vi "classifier.vi"(5 "existingTarget":bool, 6 "ImageSize":cluster{"Width":u32, "Height":u32}, 7 "targetCount":i32, 8 "input array":T2(array[cluster]), 9 "data":string, 10 "InitialValues":i32[](array[numeric]), 11 "Image In":T1(plugin-control)) -> (0 "output array":T2(array[cluster]))   [LabVIEW 2014]
uses:
  <vilib>/vision/Image Controls.llb/IMAQ Image.ctl
  <vilib>/vision/NI_Vision_Development_Module.lvlib
panel:
  out "cancelled?":bool=TRUE
  out "index":u32
  in  "numLocations":i32
  out "pitch":dbl
  out "roll":dbl
  out "yaw":dbl
  out "aircraftAltitude":dbl
  out "aircraftLongitude":dbl format="%#_10g"
  out "aircrftLatitude":dbl format="%#_10g"
  out "dragStart":cluster{"X":i32, "Y":i32}
  out "state":i32
  in  "Longitude":dbl format="%#_10g"
  in  "Latitude":dbl format="%#_10g"
  in  "changeOrientation":bool
  in  "Orientation":u16(ring) items=["North", "North-East", "East", "South-East", "South", "South-West", "West", "North-West"]
  in  "done":bool
  in  "Alphanumeric Color":string
  in  "Alphanumeric":string
  in  "Background Color":string
  in  "Shape":string
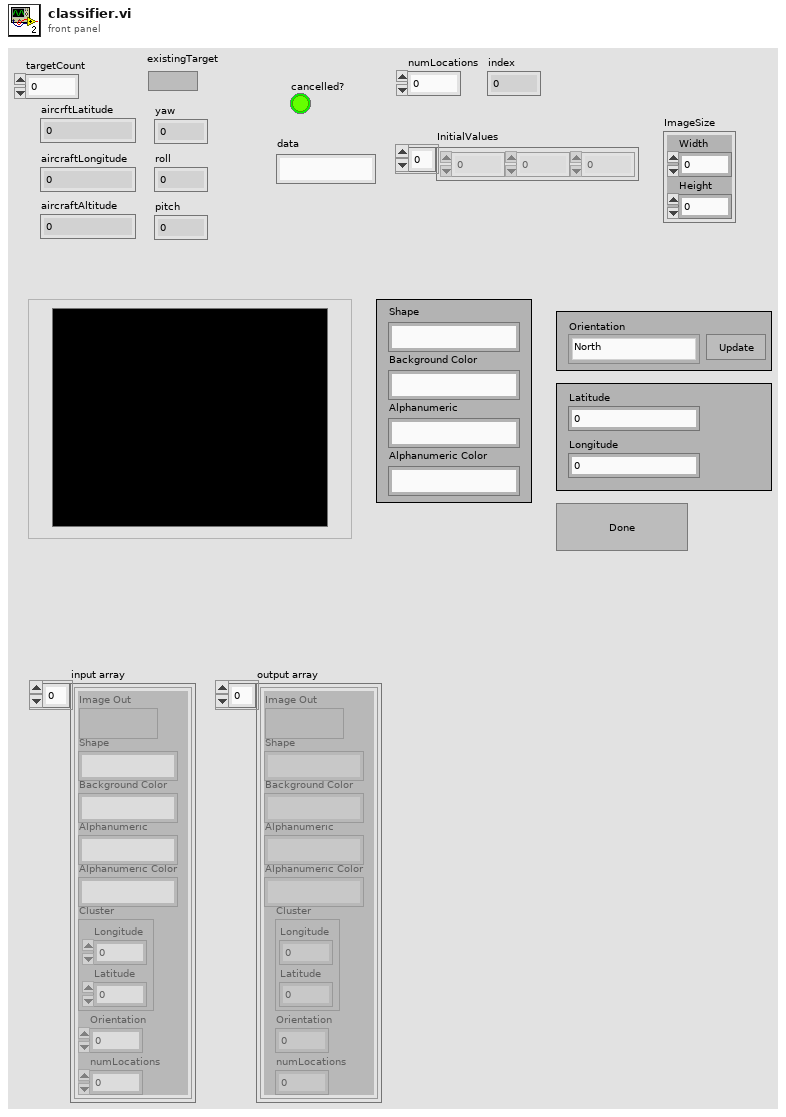
[diagram p1: front panel]
types:
  T1 = typedef "IMAQ Image.ctl" = refnum<image>
  T2 = cluster{"Image Out":T1, "Shape":string, "Background Color":string, "Alphanumeric":string, "Alphanumeric Color":string, "Cluster":cluster{"Longitude":dbl, "Latitude":dbl}, "Orientation":u16, "numLocations":i32}[]
  T3 = cluster{"Global Rectangle":i32[], "Contours":cluster{"Contour Type":u32, "ROI Type":u32, "Points":i32[]}[]}
  T4 = cluster{"Image Out":T1, "Shape":string, "Background Color":string, "Alphanumeric":string, "Alphanumeric Color":string, "Cluster":cluster{"Longitude":dbl, "Latitude":dbl}, "Orientation":u16, "numLocations":i32}
  T5 = typedef "Image Type" = u32
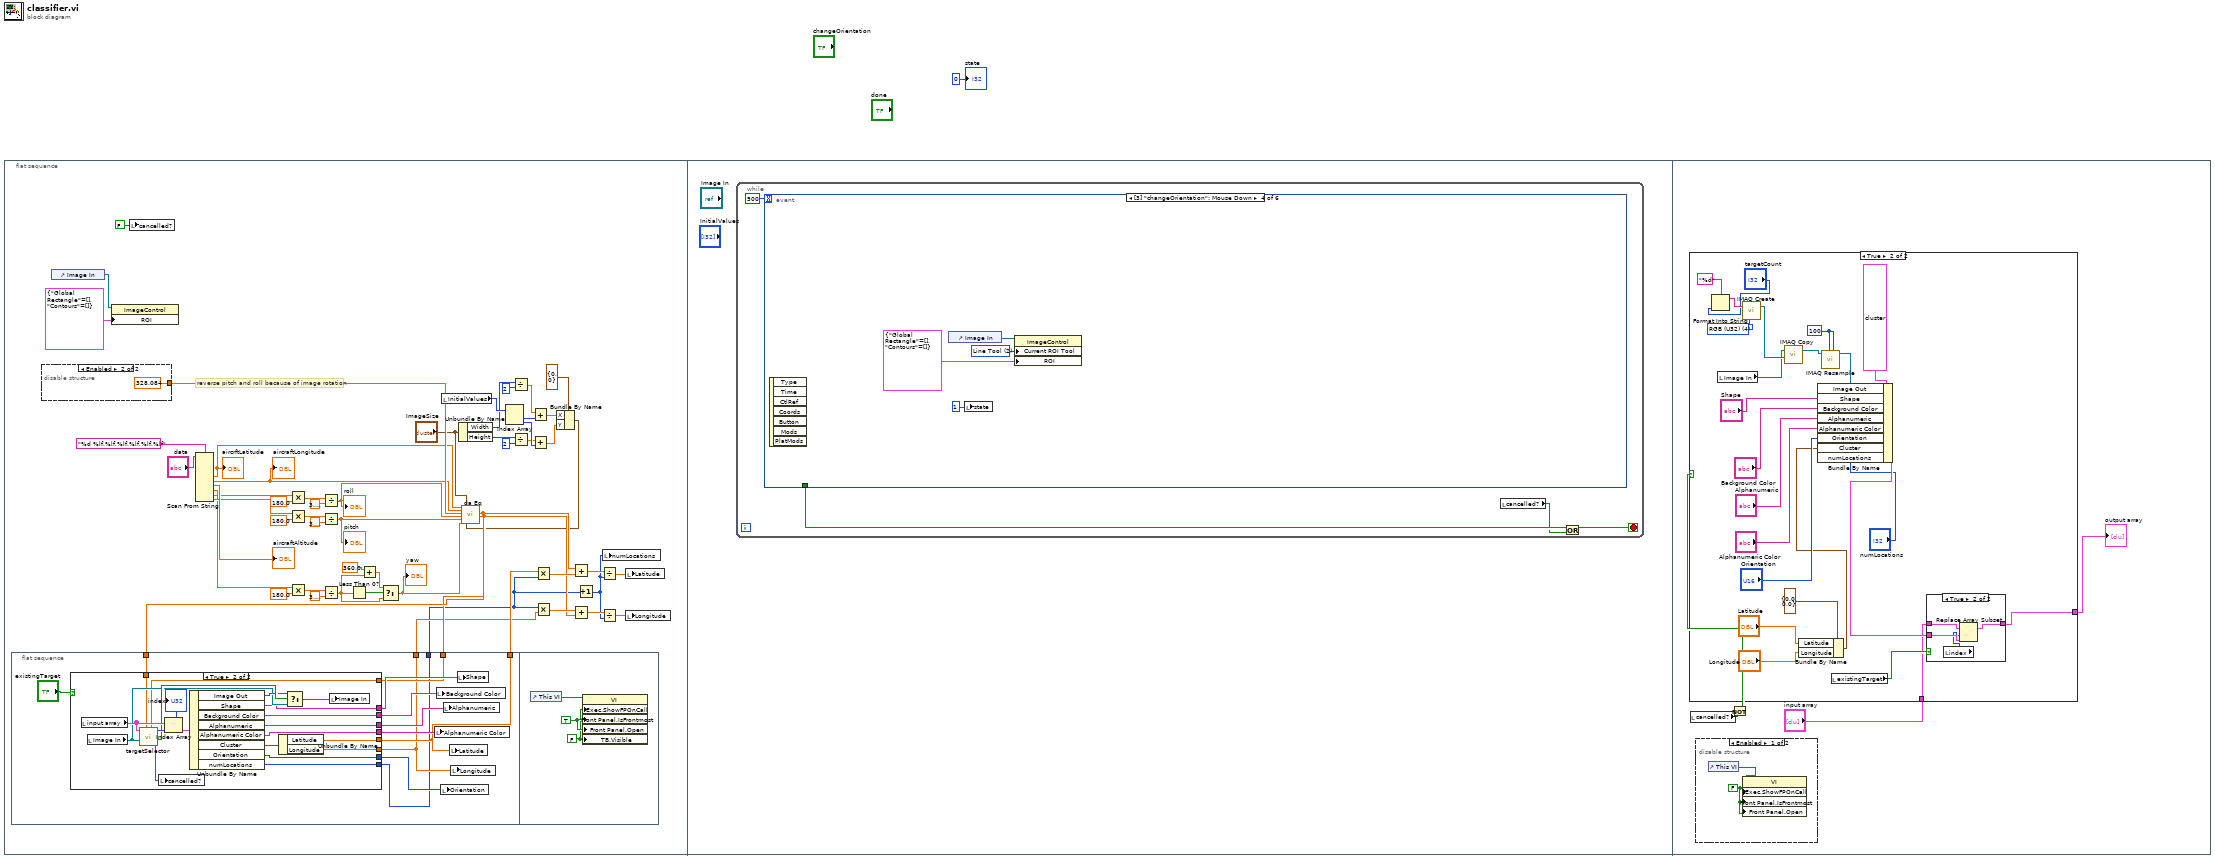
[diagram p0: block diagram]
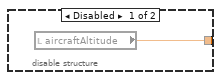
[diagram p2: hidden frame]
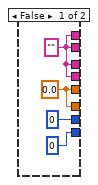
[diagram p3: hidden frame]
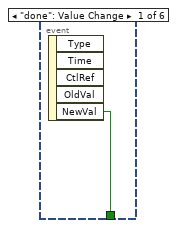
[diagram p4: hidden frame]
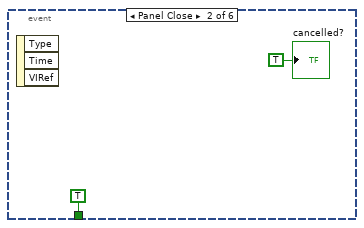
[diagram p5: hidden frame]
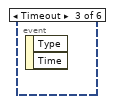
[diagram p6: hidden frame]
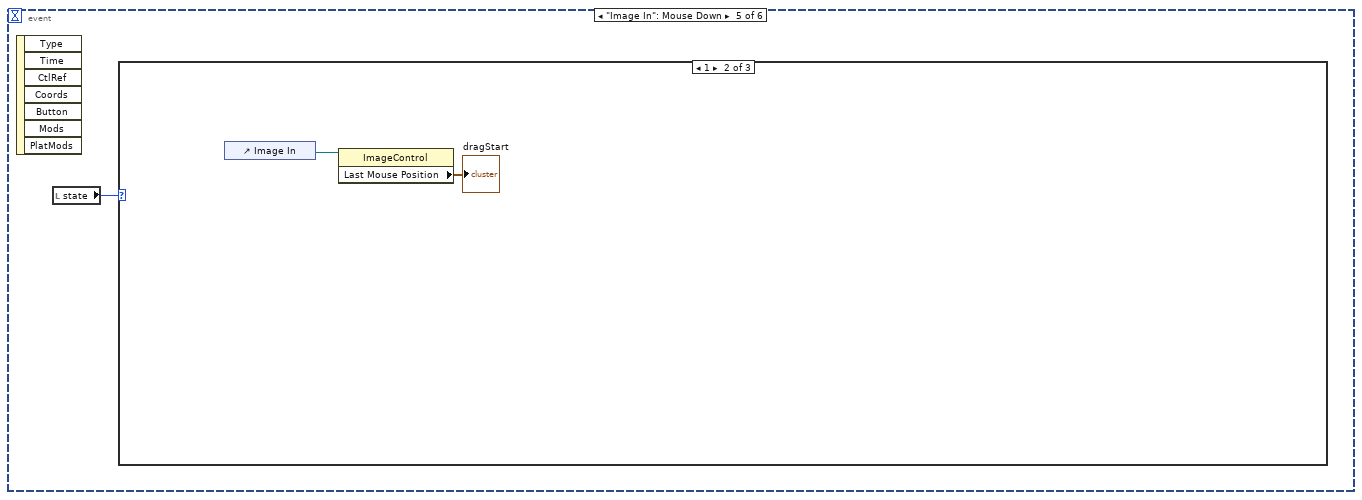
[diagram p7: hidden frame]
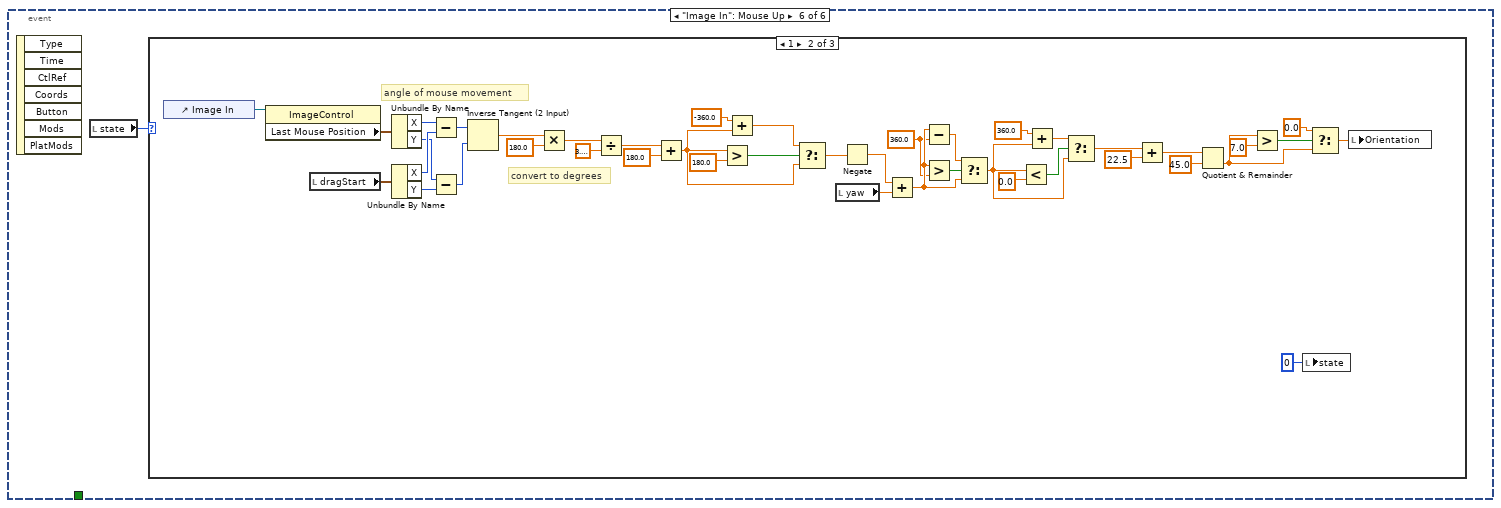
[diagram p10: hidden frame]
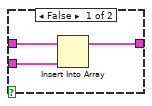
[diagram p14: hidden frame]
diagram:
  n1 = flat-sequence {
    frame #0 {
      # "reverse pitch and roll because of image rotation"
      n2 = flat-sequence {
        tunnel: w8 -> [w62]
        tunnel: w7 -> [w61]
        tunnel: [w60] -> w4
        tunnel: [w59] -> w3
        tunnel: [w58] -> w2
        frame #0 {
          n3 = case shown="True" "existingTarget" {
            tunnel: [w72 w84] -> w67
            tunnel: [w72 w83] -> w66
            tunnel: [w72 w82] -> w65
            tunnel: [w72 w81] -> w64
            tunnel: [w71 w79] -> w60
            tunnel: [w71 w78] -> w59
            tunnel: [u16 0 ("Orientation") w77] -> w63
            tunnel: [0 ("numLocations") w76] -> w58
            tunnel: w62 -> [_ w75]
            tunnel: w61 -> [_ w74]
            frame False {
              w71 = 0.0 ("Latitude")
              w72 = "" ("Shape")
            }
            frame True {
              n4 = local read "input array"() -> (w91:T2)
              n5 = local read "Image In"() -> (w86:T1)
              n6 = call "targetSelector.vi"("Longitude"=w74, "Latitude"=w75, "New Target"=w86, "Existing Targets"=w91) -> ("cancelled"=w73:bool, "imageSelect 2"=w88:bool, "index"=w90:u32)  [unwired: 5 in]
              "index" <- w90
              n7 = local write "cancelled?"(w73) -> ()
              n8 = Index Array(array=w91, index=w90) -> (element=w89:T4)
              n9 = Unbundle By Name(w89) -> ("Image Out"=w87:T1, "Shape"=w84:string, "Background Color"=w83:string, "Alphanumeric"=w82:string, "Alphanumeric Color"=w81:string, "Cluster"=w80:cluster{"Longitude":dbl, "Latitude":dbl}, "Orientation"=w77:u16, "numLocations"=w76:i32)
              n10 = Unbundle By Name(w80) -> ("Latitude"=w79:dbl, "Longitude"=w78:dbl)
              n11 = Select(t=w87, s=w88, f=w86) -> (s? t:f=w85:T1)
              n12 = local write "Image In"(w85) -> ()
            }
          }
          n13 = local write "Alphanumeric Color"(w64) -> ()
          n14 = local write "Background Color"(w66) -> ()
          n15 = local write "Orientation"(w63) -> ()
          n16 = local write "Alphanumeric"(w65) -> ()
          n17 = local write "Latitude"(w60) -> ()
          n18 = local write "Longitude"(w59) -> ()
          n19 = local write "Shape"(w67) -> ()
        }
        frame #1 {
          w92 = FALSE ("Tool Bar:Visible")
          w94 = TRUE ("Execution:Show Front Panel On Call")
          n20 = control-ref of="This VI"() -> (w93:refnum<vi>)
          n21 = property class="VI"(reference=w93, "Exec.ShowFPOnCall"=w92, "Front Panel.IsFrontmost"=w94, "Front Panel.Open"=w94, "TB.Visible"=w92) -> ()  [unwired: 1 in, 2 out]
        }
      }
      n22 = disable-structure shown="Enabled" {
        disable-tunnel: [w56 328.084 ("Plane Height (ft)")] -> w33
        frame Disabled {
          n23 = local read "aircraftAltitude"() -> (w56:dbl)
        }
        frame Enabled {
        }
      }
      n24 = control-ref of="Image In"() -> (w36:refnum<vi>)
      n25 = property class="ImageControl"(reference=w36, "ROI"=T3 {"Global Rectangle"=[], "Contours"=[]}) -> ()  [unwired: 1 in, 2 out]
      n26 = local write "cancelled?"(FALSE ("cancelled?")) -> ()
      n27 = Scan From String(format string="%d %lf,%lf,%lf,%lf,%lf,%lf", input string="data") -> (output 2=w17:dbl, output 3=w16:dbl, output 4=→"aircraftAltitude":dbl, output 5=w45:dbl, output 6=w41:dbl, output 7=w49:dbl)  [unwired: 10 in, 3 out]
      "aircrftLatitude" <- w17
      "aircraftLongitude" <- w16
      n28 = Multiply(x=w41, y=180.0) -> (x*y=w43:dbl)
      n29 = Multiply(x=w49, y=180.0) -> (x*y=w51:dbl)
      n30 = Multiply(x=w45, y=180.0) -> (x*y=w47:dbl)
      n31 = Divide(x=w43, y=3.141592653589793) -> (x/y=w20:dbl)
      "roll" <- w20
      n32 = Divide(x=w51, y=3.141592653589793) -> (x/y=w19:dbl)
      "pitch" <- w19
      n33 = Divide(x=w47, y=3.141592653589793) -> (x/y=w39:dbl)
      n34 = Less Than 0?(x=w39) -> (x < 0?=w40:bool)
      n35 = Add(x=360.0, y=w39) -> (x+y=w37:dbl)
      n36 = Select(t=w37, s=w40, f=w39) -> (s? t:f=w18:dbl)
      "yaw" <- w18
      n37 = local read "InitialValues"() -> (w30:i32[])
      n38 = Unbundle By Name("ImageSize") -> ("Width"=w14:u32, "Height"=w13:u32)
      n39 = Index Array(array=w30) -> (element #1=w29:i32, element #2=w28:i32)  [unwired: 2 in]
      n40 = Divide(x=w14, y=u32 2) -> (x/y=w10:dbl)
      n41 = Divide(x=w13, y=u32 2) -> (x/y=w9:dbl)
      n42 = Add(x=w10, y=w29) -> (x+y=w32:dbl)
      n43 = Add(x=w9, y=w28) -> (x+y=w31:dbl)
      n44 = Multiply(x=w4, y=w2) -> (x*y=w27:dbl)
      n45 = Multiply(x=w2, y=w3) -> (x*y=w26:dbl)
      n46 = Bundle By Name(cluster=cluster{"X":i32, "Y":i32} {"X"=0, "Y"=0} ("Last Mouse Position:All Elements"), "X"=w32, "Y"=w31) -> (w5:cluster{"X":i32, "Y":i32})
      n47 = call "da Eq.vi"("Plane Lat"=w17, "Plane Lon"=w16, "Plane Height (ft)"=w33, "Plane Roll"=w20, "Plane Pitch"=w19, "Plane Heading"=w18, "Displayed Image:Size:All Elements"="ImageSize", "Last Mouse Position:All Elements"=w5) -> ("Latitude"=w8:dbl, "Longitude"=w7:dbl)  [unwired: 10 in]
      n48 = Add(x=w8, y=w27) -> (x+y=w24:dbl)
      n49 = Add(x=w26, y=w7) -> (x+y=w25:dbl)
      n50 = Increment(x=w2) -> (x+1=w23:i32)
      n51 = Divide(x=w24, y=w23) -> (x/y=w22:dbl)
      n52 = Divide(x=w25, y=w23) -> (x/y=w21:dbl)
      n53 = local write "numLocations"(w23) -> ()
      n54 = local write "Latitude"(w22) -> ()
      n55 = local write "Longitude"(w21) -> ()
    }
    frame #1 {
      n56 = while {
        stop <- w96 stop-if-true
        n57 = event shown="[3] \"changeOrientation\": Mouse Down" {
          selector: _ -> [_ _ _ _ _ _]
          dyn-events: _ -> [_ _ _ _ _ _]
          timeout: 500 -> [_ _ _ _ _ _]
          tunnel: [w99 TRUE ("NewVal") _ _ _ _] -> w98
          event "done": Value Change {
            n58 = event-data() -> ("NewVal"=w99:bool)  [unwired: 1 in, 4 out]
          }
          event Panel Close {
            n59 = event-data() -> ()  [unwired: 1 in, 3 out]
            "cancelled?" <- TRUE
          }
          event Timeout {
            n60 = event-data() -> ()  [unwired: 1 in, 2 out]
          }
          event "changeOrientation": Mouse Down {
            w104 = u32 2 items=["Zoom Tool"=8, "Selection Tool"=0, "Pan Tool"=9, "Point Tool"=1, "Line Tool"=2, "Rectangle Tool"=3, "Rotated Rectangle Tool"=12, "Polyline Tool"=10, "Polygon Tool"=5, "Freehand Tool"=11, "Closed Freehand Tool"=6, "Ellipse Tool"=4, "Annulus Tool"=7] ("Current ROI Tool")
            n61 = event-data() -> ()  [unwired: 1 in, 7 out]
            n62 = control-ref of="Image In"() -> (w105:refnum<vi>)
            n63 = local write "state"(1 ("state")) -> ()
            n64 = property class="ImageControl"(reference=w105, "Current ROI Tool"=w104, "ROI"=T3 {"Global Rectangle"=[], "Contours"=[]}) -> ()  [unwired: 1 in, 2 out]
          }
          event "Image In": Mouse Down {
            n65 = event-data() -> ()  [unwired: 1 in, 7 out]
            n66 = local read "state"() -> (w106:i32)
            n67 = case shown="1" w106 {
              frame 0, Default {
              }
              frame 1 {
                n68 = control-ref of="Image In"() -> (w108:refnum<vi>)
                n69 = property class="ImageControl"(reference=w108) -> ("Last Mouse Position"=→"dragStart":cluster{"X":i32, "Y":i32})  [unwired: 1 in, 2 out]
              }
              frame 2 {
              }
            }
          }
          event "Image In": Mouse Up {
            n70 = event-data() -> ()  [unwired: 1 in, 7 out]
            n71 = local read "state"() -> (w109:i32)
            n72 = case shown="1" w109 {
              frame 0, Default {
              }
              frame 1 {
                w127 = 360.0 ("y")
                # "convert to degrees"
                # "angle of mouse movement"
                n73 = control-ref of="Image In"() -> (w145:refnum<vi>)
                n74 = property class="ImageControl"(reference=w145) -> ("Last Mouse Position"=w144:cluster{"X":i32, "Y":i32})  [unwired: 1 in, 2 out]
                n75 = local read "dragStart"() -> (w143:cluster{"X":i32, "Y":i32})
                n76 = Unbundle By Name(w144) -> ("X"=w142:i32, "Y"=w139:i32)
                n77 = Unbundle By Name(w143) -> ("X"=w141:i32, "Y"=w140:i32)
                n78 = Subtract(x=w142, y=w141) -> (x-y=w151:i32)
                n79 = Subtract(x=w139, y=w140) -> (x-y=w150:i32)
                n80 = Inverse Tangent (2 Input)(1:w150, 2:w151) -> (0:w149:dbl)
                n81 = Multiply(x=w149, y=180.0) -> (x*y=w147:dbl)
                n82 = Divide(x=w147, y=3.141592653589793) -> (x/y=w138:dbl)
                n83 = Add(x=w138, y=180.0) -> (x+y=w134:dbl)
                n84 = Greater?(x=w134, y=180.0) -> (0:w135:bool)
                n85 = Add(x=-360.0, y=w134) -> (x+y=w132:dbl)
                n86 = Select(t=w132, s=w135, f=w134) -> (s? t:f=w131:dbl)
                n87 = local read "yaw"() -> (w130:dbl)
                n88 = Negate(x=w131) -> (-x=w125:dbl)
                n89 = Add(x=w125, y=w130) -> (x+y=w128:dbl)
                n90 = Subtract(x=w128, y=w127) -> (x-y=w126:dbl)
                n91 = Greater?(x=w128, y=w127) -> (0:w129:bool)
                n92 = Select(t=w126, s=w129, f=w128) -> (s? t:f=w122:dbl)
                n93 = Less?(x=w122, y=0.0) -> (x < y?=w123:bool)
                n94 = Add(x=360.0, y=w122) -> (x+y=w120:dbl)
                n95 = Select(t=w120, s=w123, f=w122) -> (s? t:f=w119:dbl)
                n96 = Add(x=w119, y=22.5) -> (x+y=w117:dbl)
                n97 = Quotient & Remainder(x=w117, y=45.0) -> (floor(x/y)=w113:dbl)  [unwired: 1 out]
                n98 = Greater?(x=w113, y=7.0) -> (0:w114:bool)
                n99 = local write "state"(0 ("state")) -> ()
                n100 = Select(t=0.0, s=w114, f=w113) -> (s? t:f=w111:dbl)
                n101 = local write "Orientation"(w111) -> ()
              }
              frame 2 {
              }
            }
          }
        }
        n102 = local read "cancelled?"() -> (w95:bool)
        n103 = Or(x=w98, y=w95) -> (x .or. y?=w96:bool)
      }
    }
    frame #2 {
      n104 = local read "cancelled?"() -> (w155:bool)
      n105 = disable-structure shown="Enabled" {
        frame Enabled {
          w189 = FALSE ("Execution:Show Front Panel On Call")
          n106 = control-ref of="This VI"() -> (w188:refnum<vi>)
          n107 = property class="VI"(reference=w188, "Exec.ShowFPOnCall"=w189, "Front Panel.IsFrontmost"=w189, "Front Panel.Open"=w189) -> ()  [unwired: 1 in, 2 out]
        }
        frame Disabled {
        }
      }
      n108 = Not(x=w155) -> (.not. x?=w154:bool)
      n109 = case shown="True" w154 {
        tunnel: [w156 w158] -> w153
        tunnel: "input array" -> [w156 w157]
        frame False {
        }
        frame True {
          w162 = 100
          w169 = T5 4 items=["Grayscale (U8)", "Grayscale (I16)", "Grayscale (SGL)", "Complex (CSG)", "RGB (U32)", "HSL (U32)", "RGB (U64)", "Grayscale (U16)"] ("Image Type")
          n110 = Format Into String(format string="%d", "targetCount") -> (resulting string=w166:string)  [unwired: 2 in, 1 out]
          n111 = local read "Image In"() -> (w167:T1)
          n112 = call "IMAQ Create"("Image Name"=w166, "Image Type"=w169) -> ("New Image"=w168:T1)  [unwired: 3 in, 1 out]
          n113 = call "IMAQ Copy"("Image Dst"=w168, "Image Src"=w167) -> ("Image Dst Out"=w163:T1)  [unwired: 4 in, 1 out]
          n114 = Bundle By Name(cluster=cluster{"Longitude":dbl, "Latitude":dbl} {"Longitude"=0.0, "Latitude"=0.0} ("Cluster"), "Latitude"="Latitude", "Longitude"="Longitude") -> (w172:cluster{"Longitude":dbl, "Latitude":dbl})
          n115 = call "IMAQ Resample"("X Resolution"=w162, "Y Resolution"=w162, "Image Src"=w163) -> ("Image Dst Out"=w161:T1)  [unwired: 7 in, 1 out]
          n116 = Bundle By Name(cluster=T4 {"Image Out"=refnum, "Shape"="", "Background Color"="", "Alphanumeric"="", "Alphanumeric Color"="", "Cluster"={"Longitude"=0.0, "Latitude"=0.0}, "Orientation"=0, "numLocations"=0} ("output cluster"), "Image Out"=w161, "Shape"="Shape", "Background Color"="Background Color", "Alphanumeric"="Alphanumeric", "Alphanumeric Color"="Alphanumeric Color", "Orientation"="Orientation", "Cluster"=w172, "numLocations"="numLocations") -> (w171:T4)
          n117 = local read "existingTarget"() -> (w159:bool)
          n118 = case shown="True" w159 {
            tunnel: w171 -> [w183 w186]
            tunnel: w157 -> [w182 w187]
            tunnel: [w181 w184] -> w158
            frame False {
              n119 = Insert Into Array(array=w182, new element=w183) -> (w181:T2)  [unwired: 1 in]
            }
            frame True {
              n120 = local read "index"() -> (w185:u32)
              n121 = Replace Array Subset(array=w187, new element=w186, index=w185) -> (w184:T2)
            }
          }
        }
      }
      "output array" <- w153
    }
  }
  "state" <- 0
